vi "Initialise object.vi"(8 "error in (no error)":errorcluster, 9 "Connection Name":string, 10 "Serial Settings":T1={"VISA resource name "="", "baud rate"=9600, "data bits"=8, "parity"=enum."None", "stop bits"=10, "flow control"=0, "Timeout"=0, "termination char\n(0xA = '\\n' = LF) "=10, "Enable Termination Character"=FALSE} {"flow control" items=["None"=0, "XON/XOFF"=1, "RTS/CTS"=2, "DTR/DSR"=4]; "stop bits" items=["1.0"=10, "1.5"=15, "2.0"=20]; "data bits" min=5 max=8 step=1; "baud rate" items=["75"=75, "110"=110, "134"=134, "150"=150, "300"=300, "600"=600, "1200"=1200, "1800"=1800, "2400"=2400, "4800"=4800, "7200"=7200, "9600"=9600, "14400"=14400, "19200"=19200, "28800"=28800, "38400"=38400, "56000"=56000, "57600"=57600, "115200"=115200, "128000"=128000, "230400"=230400]}, 11 "Serial_comms in":refnum<class "Serial_comms.lvclass">) -> (0 "error out":errorcluster, 3 "Serial_comms out":refnum<class "Serial_comms.lvclass">)   [LabVIEW 2020, in "Serial_comms.lvlib" / "Serial_comms.lvclass"]
uses:
  Serial_comms.lvclass
  Serial_settings.ctl
  Serial_comms.lvclass/Serial_comms.ctl
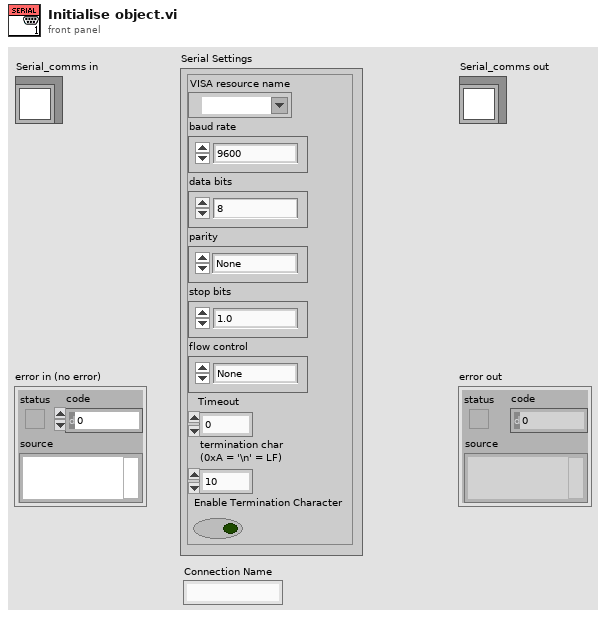
[diagram p1: front panel]
types:
  T1 = typedef "Serial_comms.lvlib/Serial_comms.lvclass/Serial_settings.ctl" = cluster{"VISA resource name ":refnum<visa-resource-name>, "baud rate":u32, "data bits":u16, "parity":enum16{"None", "Odd", "Even", "Mark", "Space"}, "stop bits":u16, "flow control":u16, "Timeout":u32, "termination char\n(0xA = '\\n' = LF) ":u8, "Enable Termination Character":bool}
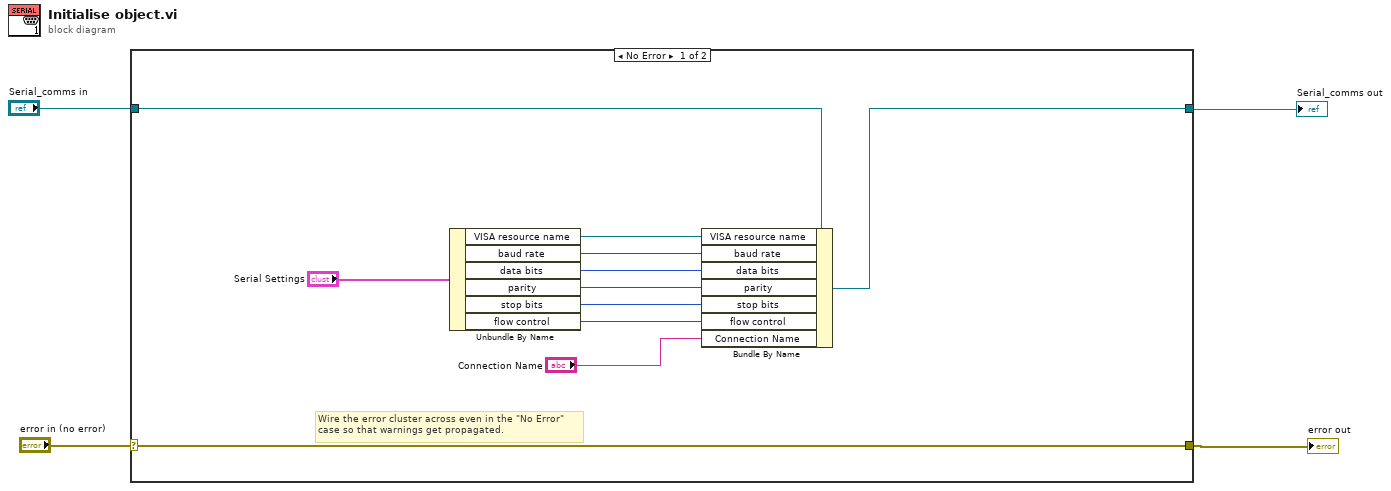
[diagram p0: block diagram]
diagram:
  n1 = case shown="No Error" "error in (no error)" {
    selector: "error in (no error)" -> [w15 w17]
    tunnel: [w15 w17] -> w3
    tunnel: [w5 w16] -> w1
    tunnel: "Serial_comms in" -> [w6 w16]
    frame No Error {
      # "Wire the error cluster across even in the \"No Error\"\ncase so that warnings get propagated."
      n2 = Unbundle By Name("Serial Settings") -> ("VISA resource name"=w14:refnum<visa-resource-name>, "baud rate"=w13:u32, "data bits"=w12:u16, "parity"=w11:enum16{"None", "Odd", "Even", "Mark", "Space"}, "stop bits"=w10:u16, "flow control"=w9:u16)
      n3 = Bundle By Name(cluster=w6, "VISA resource name"=w14, "baud rate"=w13, "data bits"=w12, "parity"=w11, "stop bits"=w10, "flow control"=w9, "Connection Name"="Connection Name") -> (w5:refnum<class "Serial_comms.lvclass">)
    }
    frame Error {
    }
  }
  "error out" <- w3
  "Serial_comms out" <- w1
